vi "Tool Data.ToolObjectsSynchronous.vi"(6 "Timeout":i32=-1, 8 "error in (no error)":errorcluster, 10 "Update Objects":T2={"Settings"={"Paths"=[], "Rectangles"=[], "Funnels"=[], "Dots"=[]}, "Data"={"Paths"=[], "Rectangles"=[], "SVGImage"=refnum, "Dots"=[], "Funnels"=[]}}, 11 "Tool Data in":refnum<class "Tool Data.lvclass">) -> (0 "error out":errorcluster, 2 "Object Updated":T1, 3 "Tool Data out":refnum<class "Tool Data.lvclass">)   [LabVIEW 2019, in "Tool Data.lvclass"]
uses:
  Tool Data.lvclass
  Typedefs/PrivateEvents--Tool Data.Update Objects.ctl
  Parse/Image/SVGImage.lvclass
  Settings/Setting Database/Typedefs/PublicEvents--Setting Database.PathsUpdated.ctl
  Settings/Path Settings/Path Settings.lvclass
  Settings/Setting Database/Typedefs/PublicEvents--Setting Database.RectanglesUpdated.ctl
  Settings/Rectangle Settings/Rectangle Settings.lvclass
  Settings/Setting Database/Typedefs/PublicEvents--Setting Database.FunnelsUpdated.ctl
  Settings/Funnel Settings/Funnel Settings.lvclass
  Settings/Setting Database/Typedefs/PublicEvents--Setting Database.DotsUpdated.ctl
  Settings/Dot Settings/Dot Settings.lvclass
  Parse/ParsePaths/Path.lvclass
  Parse/Rectangle/Rectangle.lvclass
  Parse/Dot/Dot.lvclass
  Typedefs/PublicEvents--Tool Data.Objects Updated.ctl
  Tool Path/Tool Path.lvclass
  Tool Funnel/Tool Funnel.lvclass
  Tool Rectangle/Tool Rectangle.lvclass
  Tool Dot/Tool Dots.lvclass
  Settings/Setting Database/Setting Database.lvclass
panel:
  out "Benchmark":u32
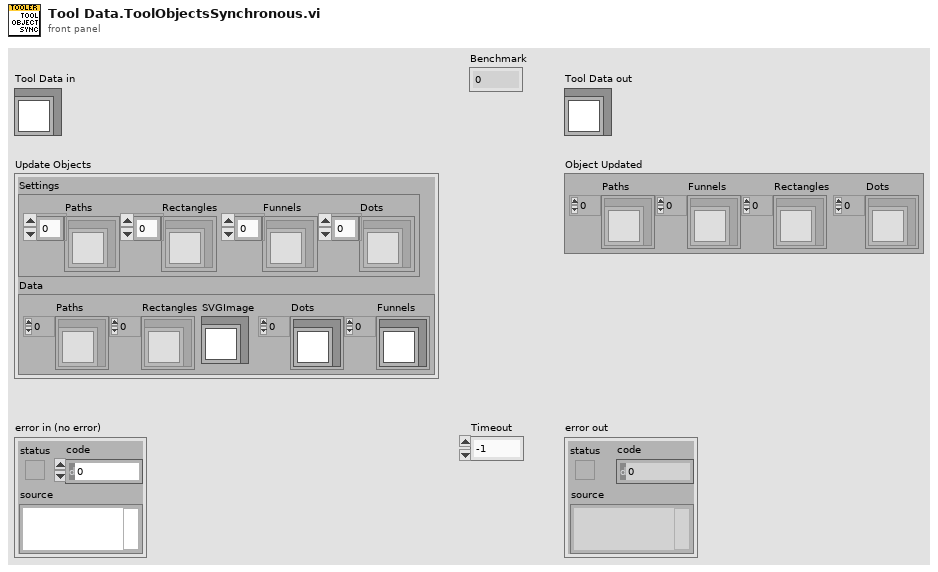
[diagram p1: front panel]
types:
  T1 = typedef "Tool Data.lvclass/PublicEvents--Tool Data.Objects Updated.ctl" = cluster{"Paths":refnum<class "Tool Path.lvclass">[], "Funnels":refnum<class "Tool Funnel.lvclass">[], "Rectangles":refnum<class "Tool Rectangle.lvclass">[], "Dots":refnum<class "Tool Dots.lvclass">[]}
  T2 = typedef "Tool Data.lvclass/PrivateEvents--Tool Data.Update Objects.ctl" = cluster{"Settings":cluster{"Paths":T3, "Rectangles":T4, "Funnels":T5, "Dots":T6}, "Data":cluster{"Paths":refnum<class "Path.lvclass">[], "Rectangles":refnum<class "Rectangle.lvclass">[], "SVGImage":refnum<class "SVGImage.lvclass">, "Dots":refnum<class "Dot.lvclass">[], "Funnels":refnum<class "Path.lvclass">[]}}
  T3 = typedef "Setting Database.lvclass/PublicEvents--Setting Database.PathsUpdated.ctl" = refnum<class "Path Settings.lvclass">[]
  T4 = typedef "Setting Database.lvclass/PublicEvents--Setting Database.RectanglesUpdated.ctl" = refnum<class "Rectangle Settings.lvclass">[]
  T5 = typedef "Setting Database.lvclass/PublicEvents--Setting Database.FunnelsUpdated.ctl" = refnum<class "Funnel Settings.lvclass">[]
  T6 = typedef "Setting Database.lvclass/PublicEvents--Setting Database.DotsUpdated.ctl" = refnum<class "Dot Settings.lvclass">[]
  T7 = typedef "Tool Data.lvclass/PublicEvents--Cluster.ctl" = cluster{"Objects Updated":refnum<user-event>}
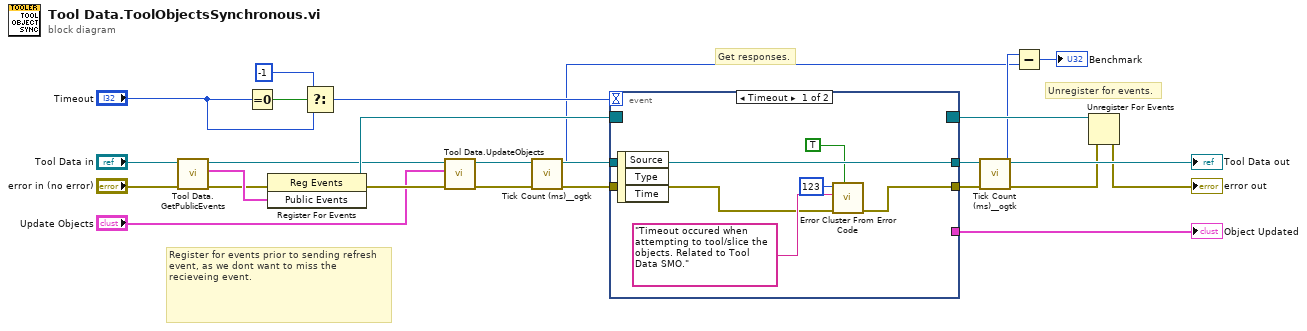
[diagram p0: block diagram]
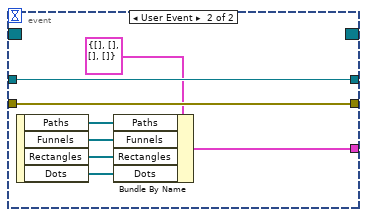
[diagram p2: hidden frame]
diagram:
  # "Unregister for events."
  # "Get responses."
  # "Register for events prior to sending refresh event, as we dont want to miss the recieveing event."
  n1 = call "Tool Data.GetPublicEvents.vi"("error in (no error)"="error in (no error)", "Tool Data"="Tool Data in") -> ("error out"=w13:errorcluster, "Public Events"=w15:T7, "Tool Data out"=w12:refnum<class "Tool Data.lvclass">)  [unwired: 7 in]
  n2 = Equal To 0?(x="Timeout") -> (x = 0?=w21:bool)
  n3 = register-events(error in=w13, w15) -> (reference out=w24:refnum<event-registration>, error out=w9:errorcluster)  [unwired: 1 in]
  n4 = Select(t=-1, s=w21, f="Timeout") -> (s? t:f=w19:i32)
  n5 = call "Tool Data.UpdateObjects.vi"("error in (no error)"=w9, "Updated Objects"="Update Objects", "Tool Data"=w12) -> ("error out"=w10:errorcluster, "Tool Data out"=w11:refnum<class "Tool Data.lvclass">)  [unwired: 7 in]
  n6 = call <userlib>:"Tick Count (ms)__ogtk.vi"("error in (no error)"=w10) -> ("error out"=w5:errorcluster, "millisecond timer value"=w2:u32)  [unwired: 9 in]
  n7 = event shown="[0] Timeout" {
    selector: w24 -> [_ _]
    dyn-events: [_ _] -> w23
    timeout: w19 -> [_ _]
    tunnel: w11 -> [w30 w38]
    tunnel: [w30 w38] -> w18
    tunnel: [w29 w37] -> w22
    tunnel: w5 -> [w25 w37]
    tunnel: [_ w31] -> w7
    event Timeout {
      n8 = event-data() -> ()  [unwired: 1 in, 3 out]
      n9 = call <vilib>:"Error Cluster From Error Code.vi"("show call chain? (False)"=TRUE, "error in (no error)"=w25, "error message (\"\")"="Timeout occured when attempting to tool/slice the objects. Related to Tool Data SMO." ("error message (\"\")"), "error code (0)"=123) -> ("error out"=w29:errorcluster)  [unwired: 5 in]
    }
    event User Event {
      n10 = event-data() -> ("Paths"=w35:refnum<class "Tool Path.lvclass">[], "Funnels"=w34:refnum<class "Tool Funnel.lvclass">[], "Rectangles"=w33:refnum<class "Tool Rectangle.lvclass">[], "Dots"=w32:refnum<class "Tool Dots.lvclass">[])  [unwired: 1 in]
      n11 = Bundle By Name(cluster=T1 {"Paths"=[], "Funnels"=[], "Rectangles"=[], "Dots"=[]} ("Objects Updated"), "Paths"=w35, "Funnels"=w34, "Rectangles"=w33, "Dots"=w32) -> (w31:T1)
    }
  }
  "Tool Data out" <- w18
  "Object Updated" <- w7
  n12 = call <userlib>:"Tick Count (ms)__ogtk.vi"("error in (no error)"=w22) -> ("error out"=w4:errorcluster, "millisecond timer value"=w3:u32)  [unwired: 9 in]
  n13 = Subtract(x=w3, y=w2) -> (x-y=→"Benchmark":u32)
  n14 = Unregister For Events(event registration refnum=w23, error in=w4) -> (error out=→"error out":errorcluster)
